vi "Menu - Add Level.vi"(10 "In":string) -> (2 "Out":string)   [LabVIEW 2019]
doc: "JSMA Module Template - Top Level UI 0.2.0.4\nRob Humfeld - Jet Engineering\nCopyright (c) 2019, Jet Engineering"
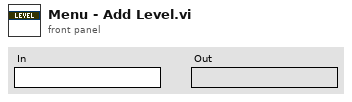
[diagram p1: front panel]
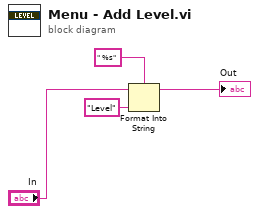
[diagram p0: block diagram]
diagram:
  n1 = Format Into String(format string=" %s", initial string="In", "Level" ("input 1")) -> (resulting string=→"Out":string)  [unwired: 1 in, 1 out]
